vi "QuerySwitchDialog.vi"() -> (0 "drop?":bool, 2 "机箱选择 2":string(combo)="A2", 3 "开关箱编号 2":string(combo)="A2")   [LabVIEW 2015]
uses:
  Global/Globalclient.vi
panel:
  in  "机箱选择":string(combo)="RF_A"
  in  "Cancel":bool
  in  "OK":bool
  in  "开关箱编号":string(combo)="1"
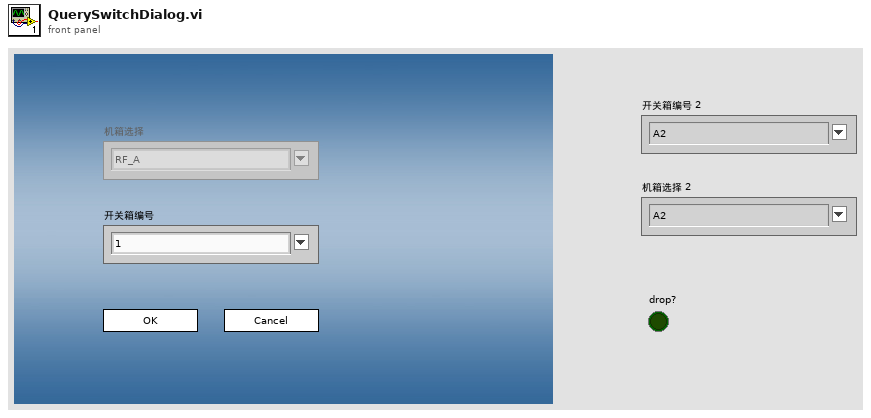
[diagram p1: front panel]
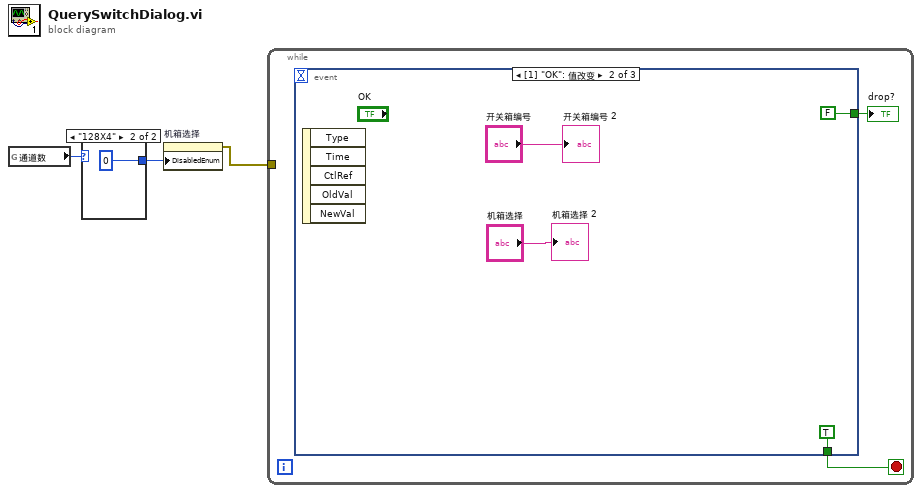
[diagram p0: block diagram]
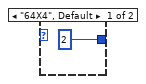
[diagram p2: hidden frame]
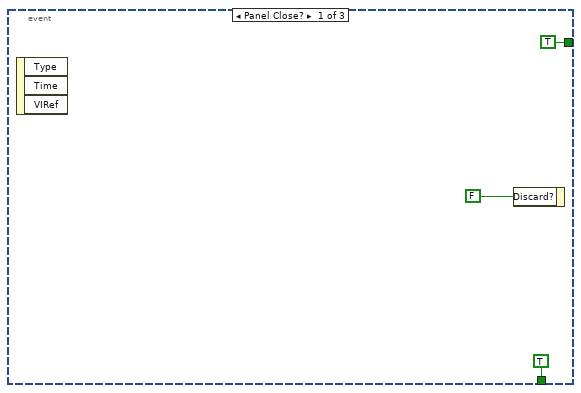
[diagram p3: hidden frame]
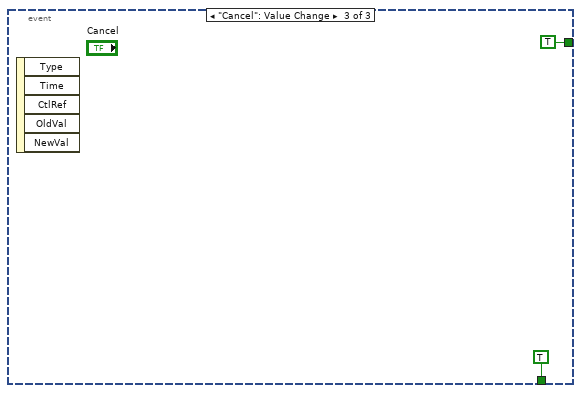
[diagram p4: hidden frame]
diagram:
  n1 = global read "Globalclient.vi" "通道数"() -> (w3:enum16{"64X4", "128X4"})
  n2 = case shown="\"128X4\"" w3 {
    tunnel: [2 0] -> w2
    frame "64X4", Default {
    }
    frame "128X4" {
    }
  }
  n3 = property on="机箱选择" class="CmbBox"("DisabledEnum"=w2) -> (error out=w1:errorcluster)  [unwired: 2 in, 1 out]
  n4 = while {
    tunnel: w1 -> [_]
    stop <- w6 stop-if-true
    n5 = event shown="[1] \"OK\": 值改变" {
      selector: _ -> [_ _ _]
      dyn-events: _ -> [_ _ _]
      timeout: _ -> [_ _ _]
      tunnel: [TRUE FALSE TRUE] -> w7
      tunnel: [TRUE TRUE TRUE] -> w6
      event Panel Close? {
        n6 = event-data() -> ()  [unwired: 1 in, 3 out]
        n7 = event-data("Discard?"=FALSE ("放弃？")) -> ()  [unwired: 1 in, 1 out]
      }
      event "OK": Value Change {
        n8 = event-data() -> ()  [unwired: 1 in, 5 out]
        "开关箱编号 2" <- "开关箱编号"
        "机箱选择 2" <- "机箱选择"
      }
      event "Cancel": Value Change {
        n9 = event-data() -> ()  [unwired: 1 in, 5 out]
      }
    }
    "drop?" <- w7
  }
